vi "Launch.vi"(7 "Common Config":T1={"Launch Timeout [ms]"=-1, "Wait For Launch Completed"=FALSE, "Front Panel State"=enum."Standard", "Close FP On Shutdown"=TRUE, "Response Channel"=refnum, "Sub Panel"=refnum}, 8 "error in (no error)":errorcluster) -> (0 "error out":errorcluster, 3 "Launch Time":timestamp)   [LabVIEW 2015, in "Task Scheduler Actor.lvclass"]
doc: "<b>Response</b> channel is used by this actor to return infomation back to the parent. Typically this input is the Request channel of the parent actor."
uses:
  Task Scheduler Actor.lvclass
  Re-use Libraries/Minimal Actor Framework/Actors/Base Actor/Actor/Common Config.ctl
  Re-use Libraries/Minimal Actor Framework/Messaging/Messenger/Messenger.lvclass
  Re-use Libraries/Minimal Actor Framework/Actors/Base Actor/Actor/Front Panel State.ctl
  API/Task Scheduler Actor API.lvclass
  Globals.vi
  Re-use Libraries/Minimal Actor Framework/Actors/Base Actor/Actor/Actor.lvclass
  Re-use Libraries/Minimal Actor Framework/Actors/Base Actor/API/Actor API.lvclass
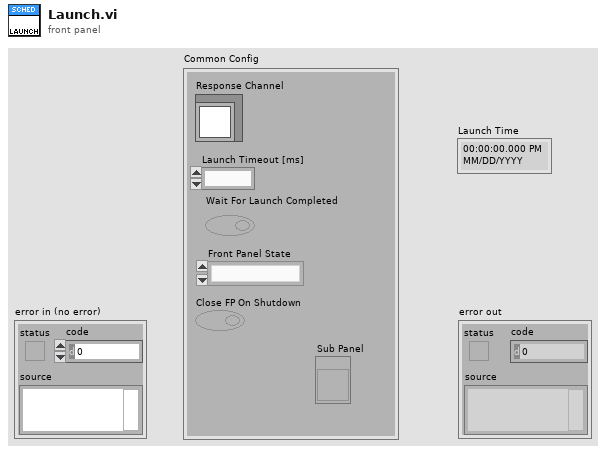
[diagram p1: front panel]
types:
  T1 = typedef "Actor.lvclass/Common Config.ctl" = cluster{"Launch Timeout [ms]":i32, "Wait For Launch Completed":bool, "Front Panel State":T2, "Close FP On Shutdown":bool, "Response Channel":refnum<class "Messenger.lvclass">, "Sub Panel":refnum<vi>}
  T2 = typedef "Actor.lvclass/Front Panel State.ctl" = enum32{"Invalid", "Standard", "Closed", "Hidden", "Minimized", "Maximized"}
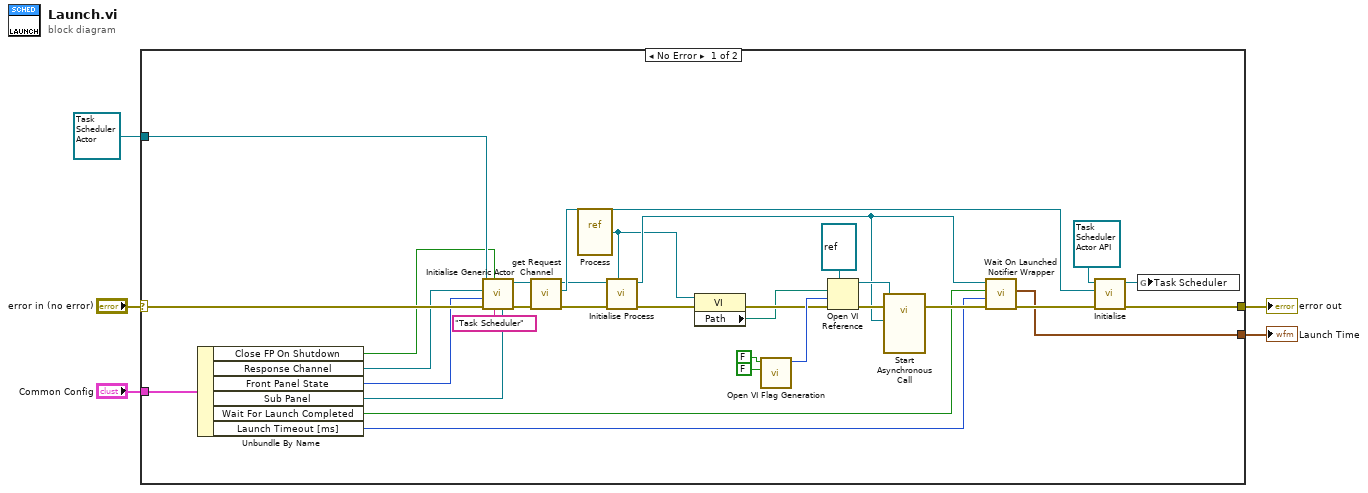
[diagram p0: block diagram]
diagram:
  n1 = case shown="No Error" "error in (no error)" {
    selector: "error in (no error)" -> [w28 w37]
    tunnel: [w27 w37] -> w5
    tunnel: refnum<class "Task Scheduler Actor.lvclass"> refnum ("Worker Test 1.lvclass") -> [w21 _]
    tunnel: [w24 _] -> w2
    tunnel: "Common Config" -> [w8 _]
    frame No Error {
      n2 = Unbundle By Name(w8) -> ("Close FP On Shutdown"=w14:bool, "Response Channel"=w13:refnum<class "Messenger.lvclass">, "Front Panel State"=w12:T2, "Sub Panel"=w11:refnum<vi>, "Wait For Launch Completed"=w10:bool, "Launch Timeout [ms]"=w9:i32)
      n3 = call-dynamic "Initialise Generic Actor.vi"("Sub Panel"=w11, "Name"="Task Scheduler", "Close FP On Shutdown (T)"=w14, "Front Panel State"=w12, "Response Channel"=w13, "Actor in"=w21) -> ("Actor out"=w29:refnum<class "Task Scheduler Actor.lvclass">)  [unwired: 4 in, 1 out]
      n4 = call "get Request Channel.vi"("error in (no error)"=w28, "Actor in"=w29) -> ("error out"=w20:errorcluster, "Request Channel"=w30:refnum<class "Messenger.lvclass">, "Actor out"=w18:refnum<class "Task Scheduler Actor.lvclass">)  [unwired: 7 in]
      n5 = vi-ref "Process.vi"() -> (w16:refnum<vi>)
      n6 = call-dynamic "Initialise Process.vi"("Process"=w16, "error in (no error)"=w20, "Actor in"=w18) -> ("error out"=w19:errorcluster, "Actor out"=w17:refnum<class "Task Scheduler Actor.lvclass">)  [unwired: 7 in]
      n7 = property class="VI"(reference=w16, error in=w19) -> (error out=w23:errorcluster, "Path"=w22:path)  [unwired: 1 out]
      n8 = call "Open VI Flag Generation.vi"("Call And Collect (F)"=FALSE, "Re-entrant (F)"=FALSE) -> ("Flags"=w36:i32)  [unwired: 9 in]
      n9 = Open VI Reference(type specifier VI Refnum (for type only)=refnum<vi> refnum, vi path=w22, options=w36, error in (no error)=w23) -> (vi reference=w32:refnum<vi>, error out=w31:errorcluster)  [unwired: 2 in]
      n10 = call-by-ref "Start Asynchronous Call"(reference=w32, error in=w31, "Worker Test 1.lvclass"=w17) -> (error out=w26:errorcluster)  [unwired: 11 in, 1 out]
      n11 = call-dynamic "Wait On Launched Notifier Wrapper.vi"("error in (no error)"=w26, "Launch Timeout [ms]"=w9, "Wait For Launch Completed"=w10, "Actor in"=w17) -> ("error out"=w25:errorcluster, "Launch Time"=w24:timestamp)  [unwired: 5 in, 1 out]
      n12 = call "Initialise.vi"("error in (no error)"=w25, "Request Channel"=w30, "Actor API in"=refnum<class "Task Scheduler Actor API.lvclass"> refnum ("Timers Manager Actor API.lvclass")) -> ("error out"=w27:errorcluster, "Actor API out"=w15:refnum<class "Task Scheduler Actor API.lvclass">)  [unwired: 7 in]
      n13 = global write "Globals.vi" "Task Scheduler"(w15) -> ()
    }
    frame Error {
    }
  }
  "error out" <- w5
  "Launch Time" <- w2
